vi "SA - Get Names and Units.vi"(0 "Nb Signals":i32, 1 "Signal IN":waveform(dbl)[](array[waveform]), 5 "error in (no error)":errorcluster) -> (15 "Signal IN":waveform(dbl)[](array[waveform]), 16 "Signal Names":string[](array[string]), 17 "Signal Units":string[](array[string]), 18 "dT Units":string[](array[string]), 19 "error out":errorcluster)   [LabVIEW 2020, in "GSwFormDSP.lvclass"]
uses:
  GSwFormDSP.lvclass
  functions/Attribute List.ctl
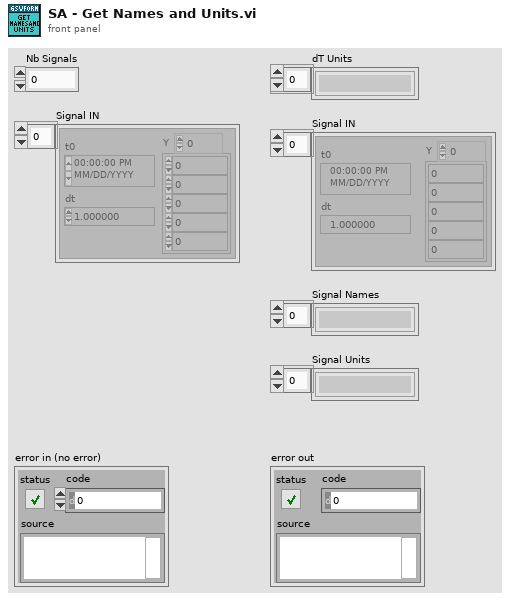
[diagram p1: front panel]
types:
  T1 = typedef "GSwFormDSP.lvclass/Attribute List.ctl" = string
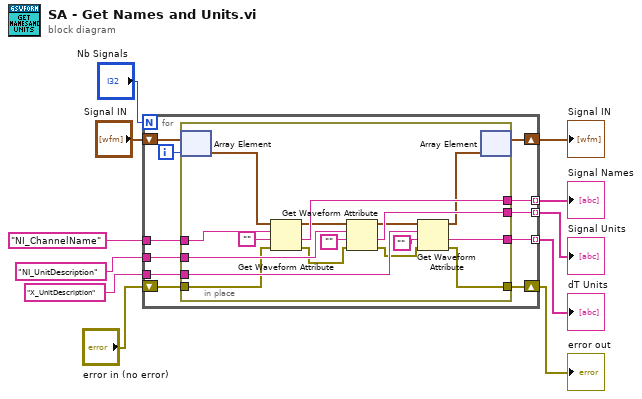
[diagram p0: block diagram]
diagram:
  n1 = for {
    N: "Nb Signals" -> [_]
    tunnel: [w21] -> w4 mode=indexing
    tunnel: [w19] -> w5 mode=indexing
    tunnel: [w17] -> w6 mode=indexing
    tunnel: T1 "NI_ChannelName" ("Attribute List") -> [w22]
    tunnel: T1 "NI_UnitDescription" ("Attribute List") -> [w20]
    tunnel: T1 "X_UnitDescription" ("Attribute List") -> [w18]
    shift-right: [w15] -> w8
    shift-left: "error in (no error)" -> [w16]
    shift-right: [w12] -> w11
    shift-left: "Signal IN" -> [w14]
    i -> [w13]
    n2 = in-place {
      in-place-border: w22 -> [w39]
      in-place-border: [w38] -> w21
      in-place-border: w20 -> [w35]
      in-place-border: [w33] -> w19
      in-place-border: w18 -> [w31]
      in-place-border: [w29] -> w17
      in-place-border: w16 -> [w28]
      in-place-border: [w25] -> w15
      n3 = in-place-array #1(w14, w13) -> (w24:waveform(dbl))
      n4 = Get Waveform Attribute(4:w28, 5:"", 6:w39, 7:w24) -> (0:w27:errorcluster, 1:w38:string, 3:w36:waveform(dbl))  [unwired: 1 out]
      n5 = Get Waveform Attribute(4:w27, 5:"", 6:w35, 7:w36) -> (0:w26:errorcluster, 1:w33:string, 3:w32:waveform(dbl))  [unwired: 1 out]
      n6 = Get Waveform Attribute(4:w26, 5:"", 6:w31, 7:w32) -> (0:w25:errorcluster, 1:w29:string, 3:w23:waveform(dbl))  [unwired: 1 out]
      n7 = in-place-array #1(w23) -> (w12:waveform(dbl)[])  [unwired: 1 out]
    }
  }
  "Signal IN" <- w11
  "error out" <- w8
  "dT Units" <- w6
  "Signal Units" <- w5
  "Signal Names" <- w4
